vi "Number to Two Bytes.vi"(9 "Fractional Precision (0)":sgl format="%#_0p", 10 "Input Value (0)":dbl) -> (1 "Byte 2":i32, 2 "Byte 1":i32)   [LabVIEW 2019, in "BK Precision 178XB Series.lvlib"]
doc: "This SubVI takes the <b>Input Value</b> and manipulates the data representation into a fractional value based on <b>Fractional Precision</b>. It then converts the value into two bytes in hexadecimal, then represented in decimal format at the output (Byte 1, Byte2).\n\nThis SubVI is used to convert set values that are in little-endian two byte format. The <b>Fractional Precision</b> is used to set the numerical representation used to convert and configure into command frame."
uses:
  BK Precision 178XB Series.lvlib
panel:
  # "(c) 2009 B&K PRECISION CORPORATION.  ALL RIGHTS RESERVED."
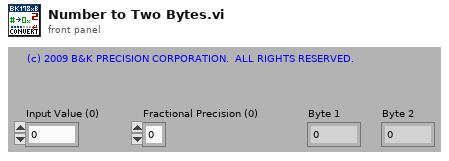
[diagram p1: front panel]
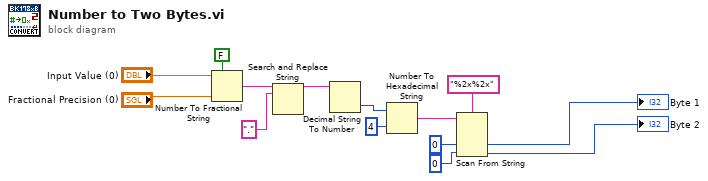
[diagram p0: block diagram]
diagram:
  n1 = Number To Fractional String(use system decimal point (T)=FALSE, number="Input Value (0)", precision (6)="Fractional Precision (0)") -> (F-format string=w12:string)  [unwired: 1 in]
  n2 = Search and Replace String(input string=w12, search string=".") -> (result string=w10:string)  [unwired: 6 in, 3 out]
  n3 = Decimal String To Number(string=w10) -> (number=w9:i32)  [unwired: 2 in, 1 out]
  n4 = Number To Hexadecimal String(1:i16 4 ("width (-)"), 2:w9) -> (0:w2:string)
  n5 = Scan From String(format string="%2x%2x", input string=w2, default 1=0 ("default value 1"), default 2=0 ("default value 2")) -> (output 1=→"Byte 1":i32, output 2=→"Byte 2":i32)  [unwired: 2 in, 3 out]
